vi "crio_FPGA_LAC_PWM_efficient.vi"() -> ()   [LabVIEW 2019]
uses:
  <vilib>/rvi/Analysis/control/PID/Typedef/niFpgaPID_PIGains.ctl
  <vilib>/rvi/Analysis/control/PID/Typedef/niFpgaPID_ManualControl.ctl
  <vilib>/rvi/Analysis/control/PID/Typedef/niFpgaPID_OutputRange.ctl
  <vilib>/rvi/Emulation/niFpgaSctlEmulationGetInTimedLoop.vi
  <vilib>/rvi/Emulation/niFpgaProcessEmulError.vi
  <vilib>/rvi/eio/common/nirviEmuTemplateMethod_errors.vi
  <vilib>/rvi/Emulation/niFpgaGetClockAttributes.vi
  <vilib>/rvi/Emulation/niFpgaEmulationReportErrorSimple.vi
  <vilib>/rvi/Emulation/niFpgaCriticalErrorInLSC.vi
  <vilib>/rvi/Analysis/control/PID/SubVIs/niFpgaPID_PIWrapper.vi
  <vilib>/eio/EIOMethodNode/EIOMethodNode.xnode
  <vilib>/eio/EIONode/EIONode.xnode
panel:
  in  "output range":T1={"output high (Inf)"=inf, "output low (-Inf)"=-inf}
  in  "LAC Lock":bool
  out "ControllerPWM Output":sgl
  in  "manual control":T2 {"manual input (0)" scale=-1.0..1.0}
  in  "setpoint":i32
  in  "gains":T3 {"proportional gain" step=0.125}
  in  "Debug: ConnectorA/DIO15":bool
  in  "Debug: ConnectorA/DIO14":bool
  in  "Encoder Debug":bool
  in  "Loop Timer DAQ":u32=1 caption="Loop Time(uSec)"
  in  "Position Reset":bool
  out "Position (Counts)":i32
  out "B":bool
  out "A":bool
  out "B'":bool
  out "A'":bool
  in  "Velocity Interval (uSec)":u32=1000
  out "Acceleration (Counts/Interval)":i32
  out "Velocity (Counts/Interval)":i32
  in  "stop":bool
  in  "DC PWM Period (us)":i16=50
  # "DRV8256 Specs:\n\n0 0: Brake Low\n1 1: Brake High\nPWM 0\n0 PWM"
  # "50 us is 20kHz"
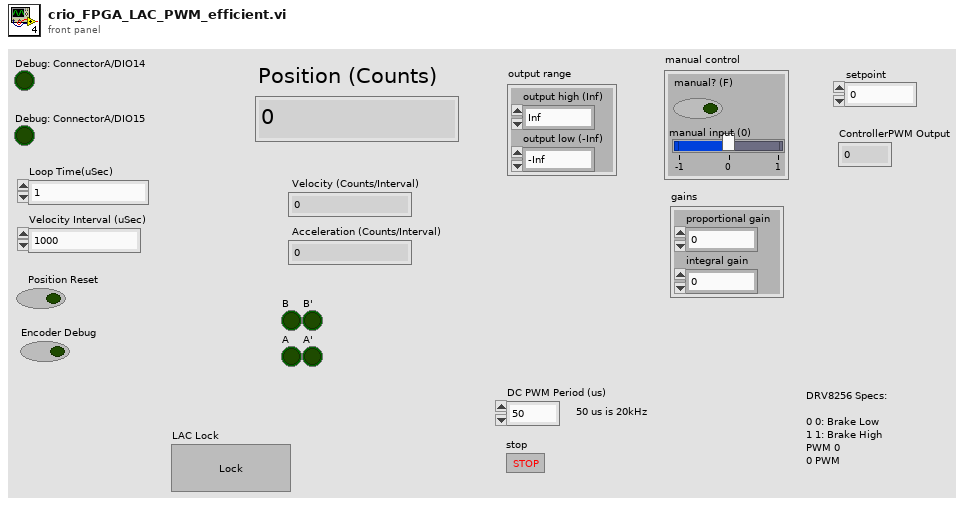
[diagram p1: front panel]
types:
  T1 = typedef "niFpgaPID_OutputRange.ctl" = cluster{"output high (Inf)":sgl, "output low (-Inf)":sgl}
  T2 = typedef "niFpgaPID_ManualControl.ctl" = cluster{"manual? (F)":bool, "manual input (0)":sgl}
  T3 = typedef "niFpgaPID_PIGains.ctl" = cluster{"proportional gain":sgl, "integral gain":sgl}
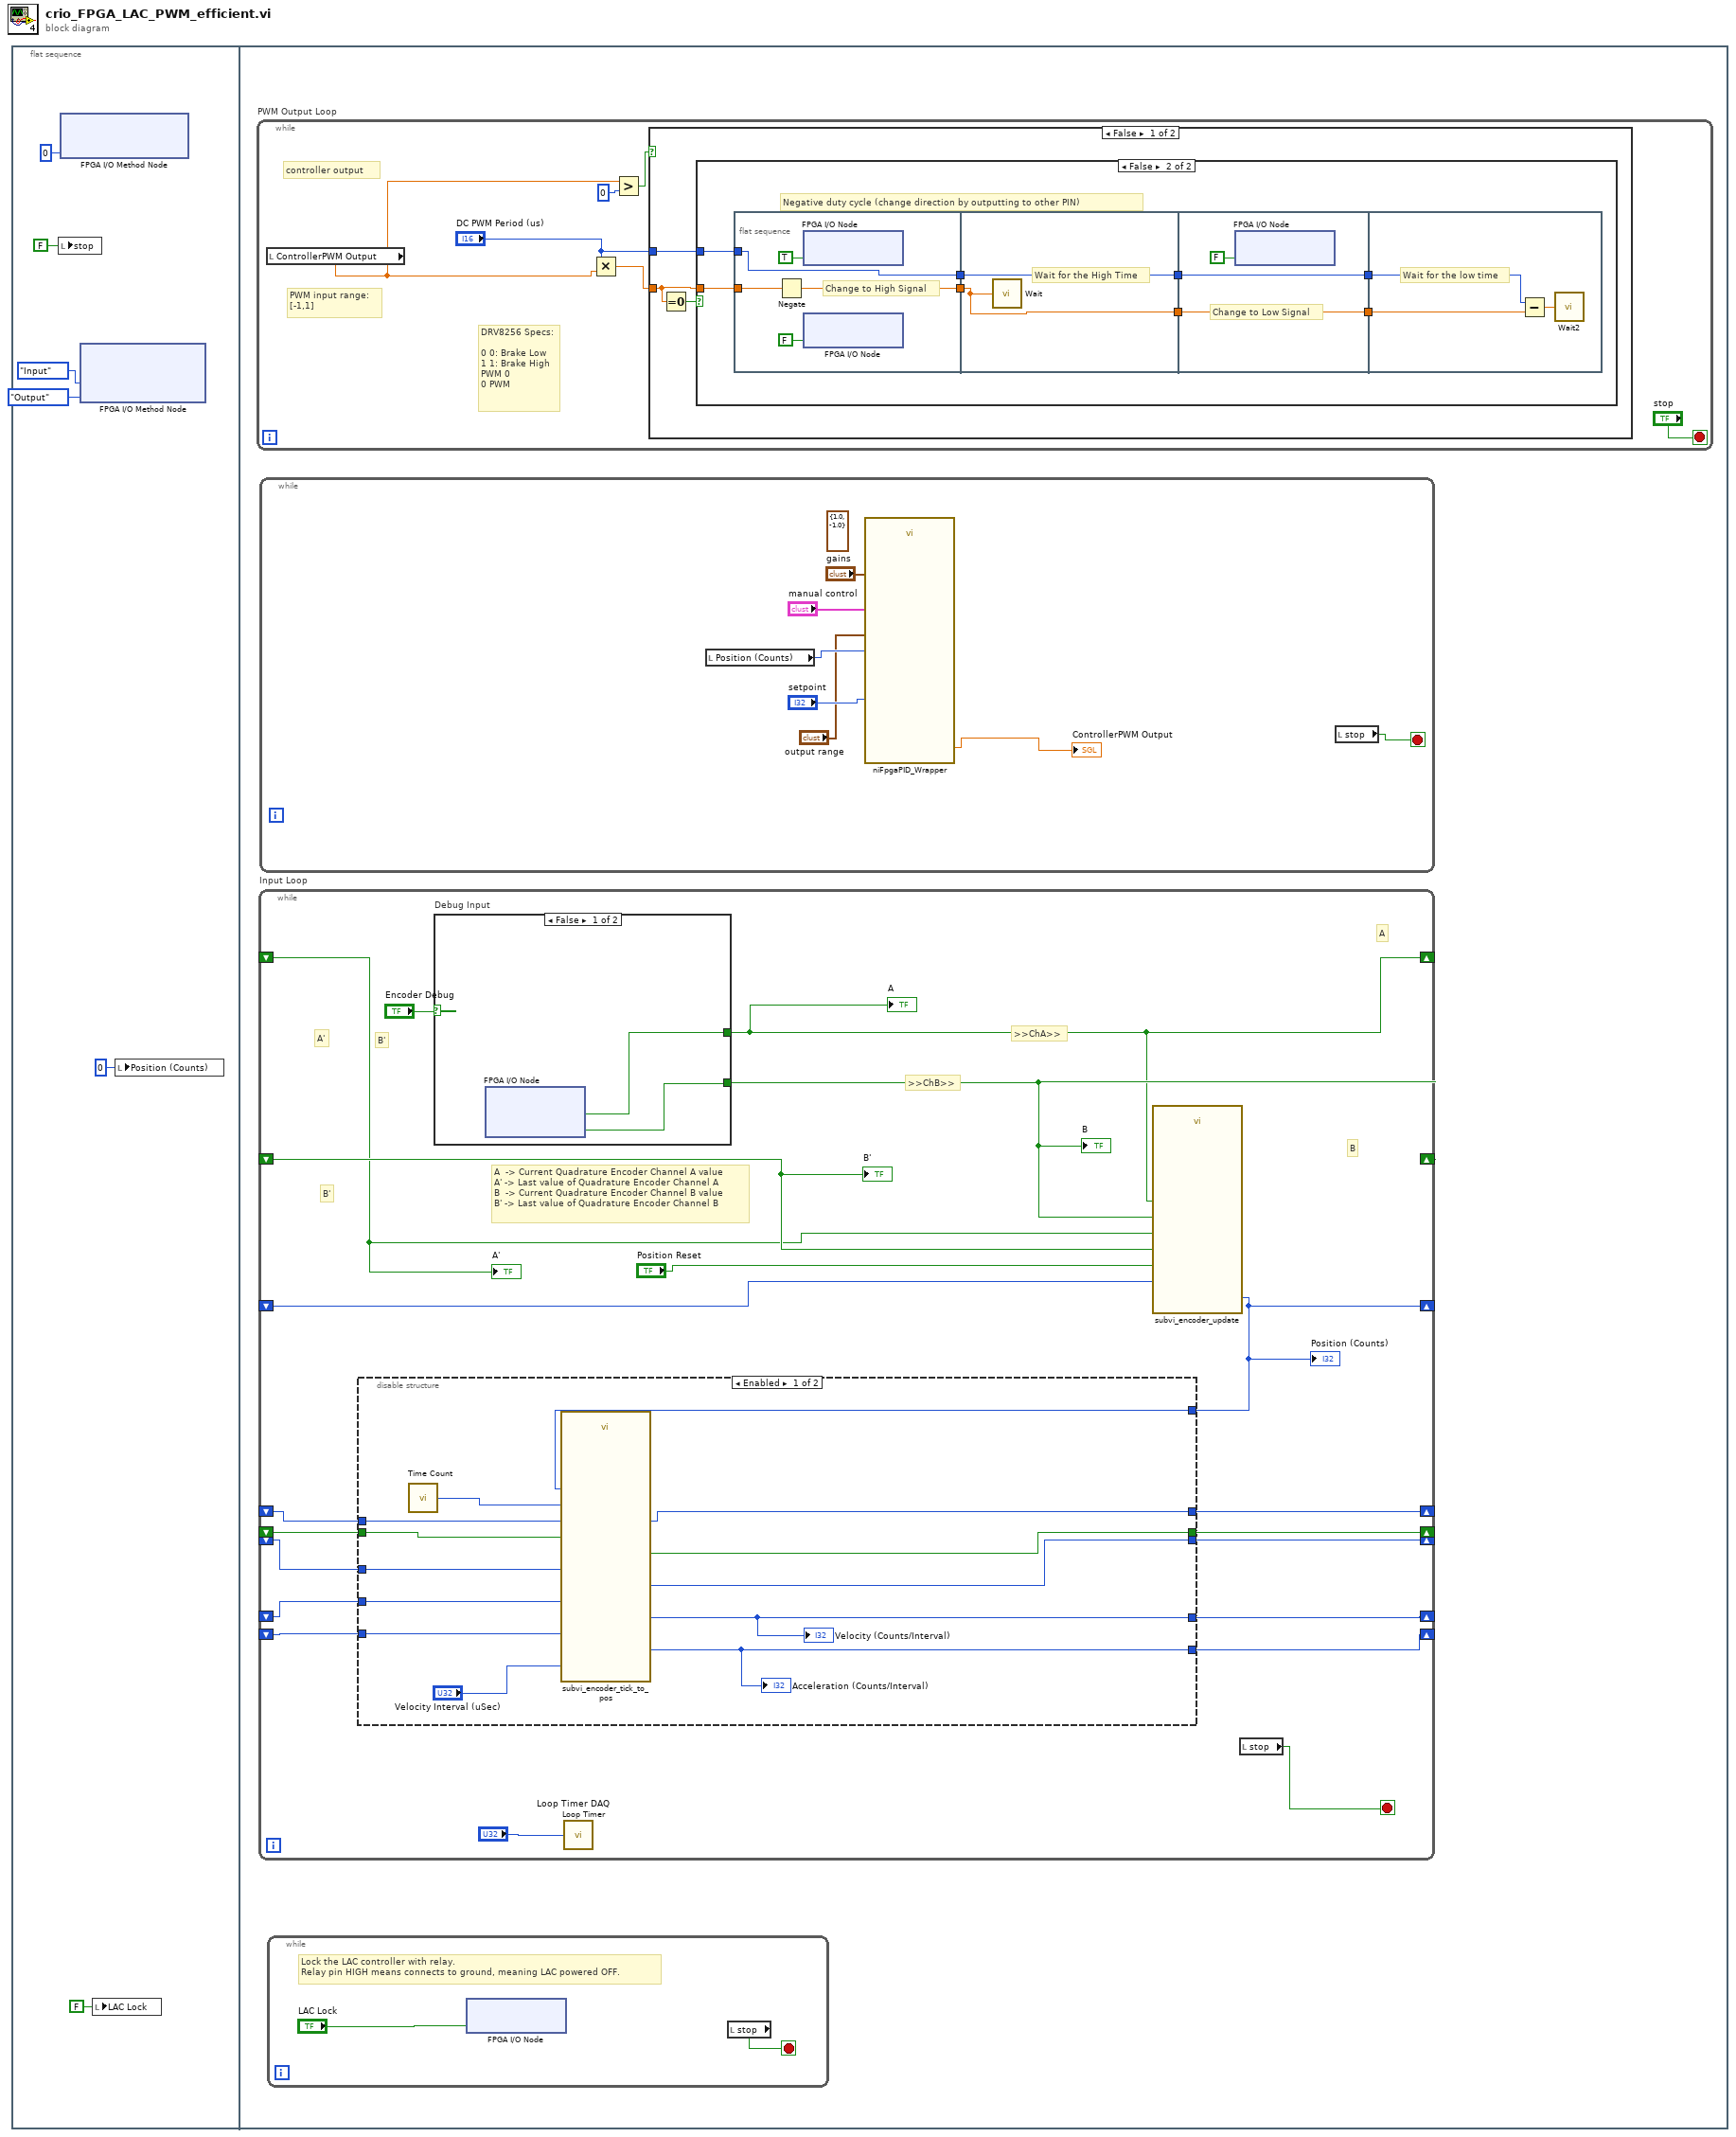
[diagram p0: block diagram]
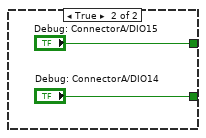
[diagram p3: hidden frame]
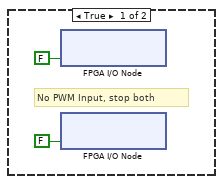
[diagram p4: hidden frame]
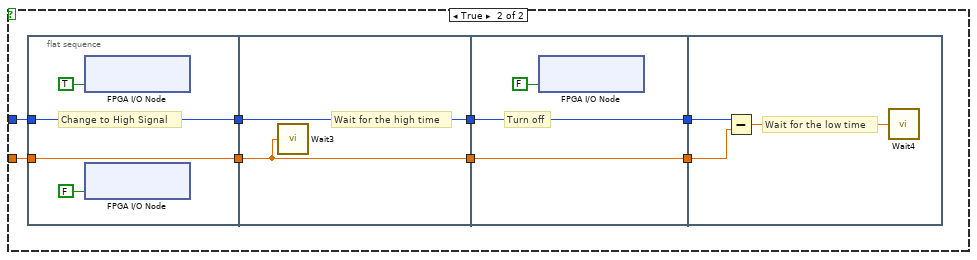
[diagram p5: hidden frame]
diagram:
  n1 = flat-sequence {
    frame #0 {
      n2 = local write "stop"(FALSE ("stop")) -> ()
      n3 = xnode "FPGA I/O Method Node"("Enable"=u8 0) -> ()  [unwired: 1 in, 1 out]
      n4 = xnode "FPGA I/O Method Node"("DIO 7:4"=enum8{"No Change", "Input", "Output"}."Input", "DIO 3:0"=enum8{"No Change", "Input", "Output"}."Output") -> ()  [unwired: 1 in, 1 out]
      n5 = local write "LAC Lock"(FALSE ("LAC Lock")) -> ()
      n6 = local write "Position (Counts)"(0 ("Position (Counts)")) -> ()
    }
    frame #1 {
      n7 = while "PWM Output Loop" {
        stop <- "stop" stop-if-true
        # "PWM input range:\n[-1,1]"
        # "DRV8256 Specs:\n\n0 0: Brake Low\n1 1: Brake High\nPWM 0\n0 PWM"
        # "controller output"
        n8 = local read "ControllerPWM Output"() -> (w53:sgl)
        n9 = Multiply(x="DC PWM Period (us)", y=w53) -> (x*y=w55:sgl)
        n10 = Greater?(x=w53, y=i16 0) -> (0:w56:bool)
        n11 = case shown="False" w56 {
          tunnel: w55 -> [w61 w92]
          tunnel: "DC PWM Period (us)" -> [w59 w91]
          frame False {
            n12 = Equal To 0?(x=w61) -> (x = 0?=w60:bool)
            n13 = case shown="False" w60 {
              tunnel: w61 -> [_ w71]
              tunnel: w59 -> [_ w64]
              frame True {
                # "No PWM Input, stop both"
                n14 = xnode "FPGA I/O Node"("Mod1/DIO2"=FALSE) -> ()  [unwired: 1 in, 1 out]
                n15 = xnode "FPGA I/O Node"("Mod1/DIO3"=FALSE) -> ()  [unwired: 1 in, 1 out]
              }
              frame False {
                # "Negative duty cycle (change direction by outputting to other PIN)"
                n16 = flat-sequence {
                  tunnel: w71 -> [w74]
                  tunnel: [w73] -> w70
                  tunnel: [w72] -> w65
                  tunnel: w64 -> [w72]
                  tunnel: w70 -> [w78]
                  tunnel: [w78] -> w69
                  tunnel: [w77] -> w66
                  tunnel: w65 -> [w77]
                  tunnel: w69 -> [w80]
                  tunnel: [w80] -> w68
                  tunnel: [w79] -> w67
                  tunnel: w66 -> [w79]
                  tunnel: w68 -> [w84]
                  tunnel: w67 -> [w83]
                  frame #0 {
                    # "Change to High Signal"
                    n17 = Negate(x=w74) -> (-x=w73:sgl)
                    n18 = xnode "FPGA I/O Node"("Mod1/DIO3"=TRUE) -> ()  [unwired: 1 in, 1 out]
                    n19 = xnode "FPGA I/O Node"("Mod1/DIO2"=FALSE) -> ()  [unwired: 1 in, 1 out]
                  }
                  frame #1 {
                    # "Wait for the High Time"
                    n20 = call "Wait"("Count(uSec)"=w78) -> ()  [unwired: 1 out]
                  }
                  frame #2 {
                    # "Change to Low Signal"
                    n21 = xnode "FPGA I/O Node"("Mod1/DIO2"=FALSE) -> ()  [unwired: 1 in, 1 out]
                  }
                  frame #3 {
                    # "Wait for the low time"
                    n22 = Subtract(x=w83, y=w84) -> (x-y=w82:sgl)
                    n23 = call "Wait2"("Count(uSec)"=w82) -> ()  [unwired: 1 out]
                  }
                }
              }
            }
          }
          frame True {
            n24 = flat-sequence {
              tunnel: w92 -> [w93]
              tunnel: w91 -> [w94]
              tunnel: [w94] -> w88
              tunnel: [w93] -> w87
              tunnel: [w98] -> w89
              tunnel: w88 -> [w98]
              tunnel: w87 -> [w97]
              tunnel: [w97] -> w86
              tunnel: [w100] -> w90
              tunnel: w89 -> [w100]
              tunnel: w86 -> [w99]
              tunnel: [w99] -> w85
              tunnel: w90 -> [w104]
              tunnel: w85 -> [w102]
              frame #0 {
                # "Change to High Signal"
                n25 = xnode "FPGA I/O Node"("Mod1/DIO2"=TRUE) -> ()  [unwired: 1 in, 1 out]
                n26 = xnode "FPGA I/O Node"("Mod1/DIO3"=FALSE ("ConnectorB/DIO9")) -> ()  [unwired: 1 in, 1 out]
              }
              frame #1 {
                # "Wait for the high time"
                n27 = call "Wait3"("Count(uSec)"=w97) -> ()  [unwired: 1 out]
              }
              frame #2 {
                # "Turn off"
                n28 = xnode "FPGA I/O Node"("Mod1/DIO2"=FALSE) -> ()  [unwired: 1 in, 1 out]
              }
              frame #3 {
                # "Wait for the low time"
                n29 = Subtract(x=w104, y=w102) -> (x-y=w103:sgl)
                n30 = call "Wait4"("Count(uSec)"=w103) -> ()  [unwired: 1 out]
              }
            }
          }
        }
      }
      n31 = while "Input Loop" {
        shift-right: [w29] -> _
        shift-left: _ -> [w32]
        shift-right: [w28] -> _
        shift-left: _ -> [w31]
        shift-right: [w24] -> _
        shift-left: _ -> [w30]
        shift-right: [w17] -> _
        shift-left: _ -> [w27]
        shift-right: [w18] -> _
        shift-left: _ -> [w26]
        shift-right: [w25] -> _
        shift-left: _ -> [w23]
        shift-right: [w22] -> _
        shift-left: _ -> [w21]
        shift-right: [w20] -> _
        shift-left: _ -> [w19]
        stop <- w16 stop-if-true
        # "B'"
        # ">>ChB>>"
        # ">>ChA>>"
        # "A'"
        # "A  -> Current Quadrature Encoder Channel A value\nA' -> Last value of Quadrature Encoder Channel A\nB  -> Current Quadrature Encoder Channel B value\nB' -> Last value of Quadrature Encoder Channel B"
        # "B'"
        # "B"
        # "A"
        n32 = case "Debug Input" shown="False" "Encoder Debug" {
          tunnel: [w50 "Debug: ConnectorA/DIO15"] -> w28
          tunnel: [w49 "Debug: ConnectorA/DIO14"] -> w29
          frame False {
            n33 = xnode "FPGA I/O Node"() -> ("Mod2/DIO2"=w50:bool, "Mod2/DIO3"=w49:bool)  [unwired: 2 in, 2 out]
          }
          frame True {
          }
        }
        "B" <- w29
        "A" <- w28
        n34 = call "Loop Timer"("Count(uSec)"="Loop Timer DAQ") -> ()  [unwired: 1 out]
        n35 = call "subvi_encoder_update.vi"("Position Reset"="Position Reset", "Tick'"=w30, "A"=w28, "B'"=w32, "A'"=w31, "B"=w29) -> ("Tick"=w24:i32)  [unwired: 5 in]
        "Position (Counts)" <- w24
        n36 = disable-structure shown="Enabled" {
          disable-tunnel: w27 -> [w47 _]
          disable-tunnel: w26 -> [w46 _]
          disable-tunnel: [w45 _] -> w25
          disable-tunnel: w24 -> [w44 _]
          disable-tunnel: w23 -> [w43 _]
          disable-tunnel: [w42 _] -> w22
          disable-tunnel: w21 -> [w41 _]
          disable-tunnel: [w40 _] -> w20
          disable-tunnel: w19 -> [w39 _]
          disable-tunnel: [w37 _] -> w18
          disable-tunnel: [w36 _] -> w17
          frame Enabled {
            n37 = call "Time Count"() -> ("Tick Count(uSec)"=w38:u32)
            n38 = call "subvi_encoder_tick_to_pos.vi"("Velocity Interval (uSec)"="Velocity Interval (uSec)", "Raw Tick"=w44, "Waited?'"=w41, "Tick Count(uSec)'"=w39, "p'"=w43, "Time Count"=w38, "a'"=w46, "v'"=w47) -> ("Waited?"=w42:bool, "Tick Count(uSec)"=w40:u32, "p"=w45:i32, "a"=w37:i32, "v"=w36:i32)  [unwired: 3 in]
            "Acceleration (Counts/Interval)" <- w37
            "Velocity (Counts/Interval)" <- w36
          }
          frame Disabled {
          }
        }
        n39 = local read "stop"() -> (w16:bool)
        "B'" <- w32
        "A'" <- w31
      }
      n40 = while {
        stop <- w15 stop-if-true
        (unwired) T1 {"output high (Inf)"=1.0, "output low (-Inf)"=-1.0} ("output range")
        n41 = local read "Position (Counts)"() -> (w14:i32)
        n42 = call-poly <vilib>:"niFpgaPID_Wrapper.vi"("setpoint"="setpoint", "process variable"=w14, "manual control"="manual control", "gains"="gains", "output range"="output range") -> ("output"=→"ControllerPWM Output":sgl)  [unwired: 8 in, 2 out]
        n43 = local read "stop"() -> (w15:bool)
      }
      n44 = while {
        stop <- w8 stop-if-true
        # "Lock the LAC controller with relay.\nRelay pin HIGH means connects to ground, meaning LAC powered OFF."
        n45 = xnode "FPGA I/O Node"("Mod8/DIO6"="LAC Lock") -> ()  [unwired: 1 in, 1 out]
        n46 = local read "stop"() -> (w8:bool)
      }
    }
  }
